vi "Send Write Stop Reason.vi"(7 "Priority":T2=enum."Normal" caption="Message Priority (Normal)", 8 "error in (no error)":errorcluster, 10 "Stop Reason":T1, 11 "Message Enqueuer in":refnum<class "Message Enqueuer.lvclass">) -> (0 "error out":errorcluster, 3 "Message Enqueuer out":refnum<class "Message Enqueuer.lvclass">)   [LabVIEW 2023, in "Iterator Actor.lvlib" / "Write Stop Reason Msg.lvclass"]
doc: "Sends the <b>Iterator Actor.lvlib:Write Stop Reason Msg.lvclass</b> message.\n\nThis message will call <b>Write Stop Reason.vi</b> on the <b>Iterator Actor.lvlib:Abstract Iterator Actor.lvclass</b> actor.\n\n<b>Write Stop Reason.vi Description</b>"
uses:
  Write Stop Reason Msg.lvclass
  Write Stop Reason Msg.lvclass/Write Stop Reason Msg.ctl
  <vilib>/ActorFramework/Message Enqueuer/Message Enqueuer.lvclass
  C:/Program Files/National Instruments/LabVIEW 2023/vi.lib/ActorFramework/Message/Message.lvclass
  C:/Projects/Iterator Actor/Abstract Iterator Actor Messages/Write Stop Reason Msg/Write Stop Reason Msg.lvclass
  <vilib>/ActorFramework/Message Enqueuer/Message Priority.ctl
  Abstract Iterator Actor/Stop Reason.ctl
  Abstract Iterator Actor/Abstract Iterator Actor.lvclass
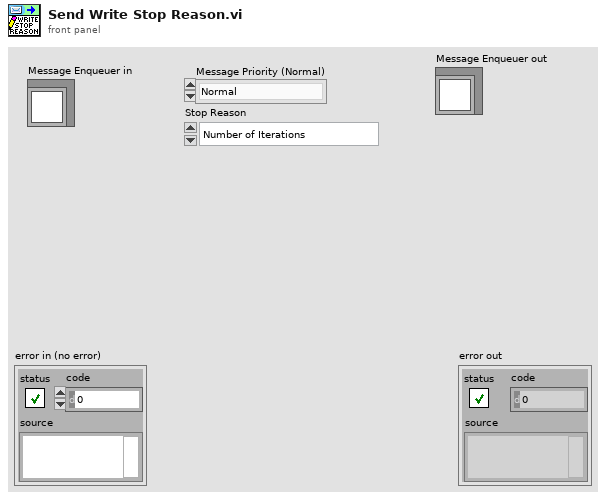
[diagram p1: front panel]
types:
  T1 = typedef "Iterator Actor.lvlib/Abstract Iterator Actor.lvclass/Stop Reason.ctl" = enum16{"Number of Iterations", "Time Elapsed", "Stopped Internally", "Stopped Externally"}
  T2 = typedef "Actor Framework.lvlib/Message Enqueuer.lvclass/Message Priority.ctl" = enum16{"Low", "Normal", "High"}
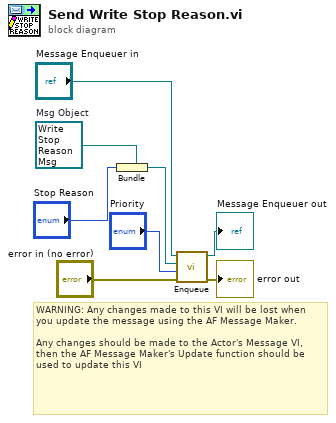
[diagram p0: block diagram]
diagram:
  w7 = refnum<class "Write Stop Reason Msg.lvclass"> refnum  # Msg Object
  # "WARNING: Any changes made to this VI will be lost when you update the message using the AF Message Maker.\n\nAny changes should be made to the Actor's Message VI, then the AF Message Maker's Update function should be used to update this VI"
  n1 = Bundle(cluster=w7, "Stop Reason") -> (w2:refnum<class "Write Stop Reason Msg.lvclass">)
  n2 = call <vilib>:"Enqueue.vi"("error in (no error)"="error in (no error)", "Message Priority (Normal)"="Priority", "Message"=w2, "Message Enqueuer in"="Message Enqueuer in") -> ("error out"=→"error out":errorcluster, "Message Enqueuer out"=→"Message Enqueuer out":refnum<class "Message Enqueuer.lvclass">)  [unwired: 6 in]
